vi "Get Result.vi"(8 "error in (no error)":errorcluster, 11 "LUnit Test Case V2 In":refnum<class "LUnit Test Case V2.lvclass">) -> (0 "error out":errorcluster, 2 "Cluster of class private data":T1, 3 "LUnit Test Case V2 Out":refnum<class "LUnit Test Case V2.lvclass">)   [LabVIEW 2020, in "LUnit Test Case V2.lvclass"]
uses:
  LUnit Test Case V2.lvclass
  Framework/Result Types/Assertion Result/Public/TypeDefs/Status.ctl
  Framework/Result Types/Assertion Result/Assertion Result.lvlib
  Framework/Result Types/Assertion Result/Public/TypeDefs/Assertion Type.ctl
  Framework/Result Types/Assertion Result/Assertion Result.ctl
  Framework/Result Types/Method Result/Method Result.ctl
  Framework/Result Types/Method Result/Method Result.lvlib
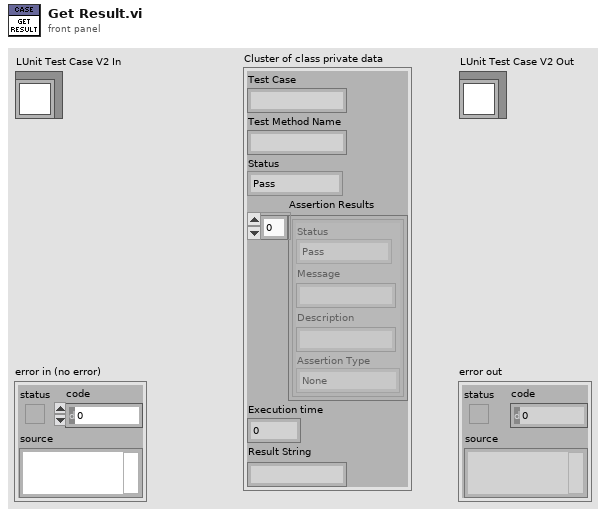
[diagram p1: front panel]
types:
  T1 = typedef "Method Result.lvlib/Method Result.ctl" = cluster{"Test Case":string, "Test Method Name":string, "Status":T2, "Assertion Results":T3[], "Execution time":dbl, "Result String":string}
  T2 = typedef "Assertion Result.lvlib/Status.ctl" = enum16{"Pass", "Fail", "Error", "Skipped", "Setup Error", "Broken", "Teardown Error"}
  T3 = typedef "Assertion Result.lvlib/Assertion Result.ctl" = cluster{"Status":T2, "Message":string, "Description":string, "Assertion Type":T4}
  T4 = typedef "Assertion Result.lvlib/Assertion Type.ctl" = enum16{"None", "Pass", "Fail", "Skip", "Pass if Equal", "Fail if Equal", "Pass if Error", "Fail if Error", "Pass if", "Fail if"}
  T5 = typedef "Result.lvlib/Result.ctl" = cluster{"Case":string, "Method":string, "Message":string, "Description":string, "Status":T6, "Result Type":T7}
  T6 = typedef "Result.lvlib/Status.ctl" = enum16{"Pass", "Fail", "Error", "Skipped", "Setup Error", "Broken", "Teardown Error"}
  T7 = typedef "Result.lvlib/Type.ctl" = enum16{"None", "Pass", "Fail", "Skip", "Pass if Equal", "Fail if Equal", "Pass if Error", "Fail if Error", "Pass if", "Fail if"}
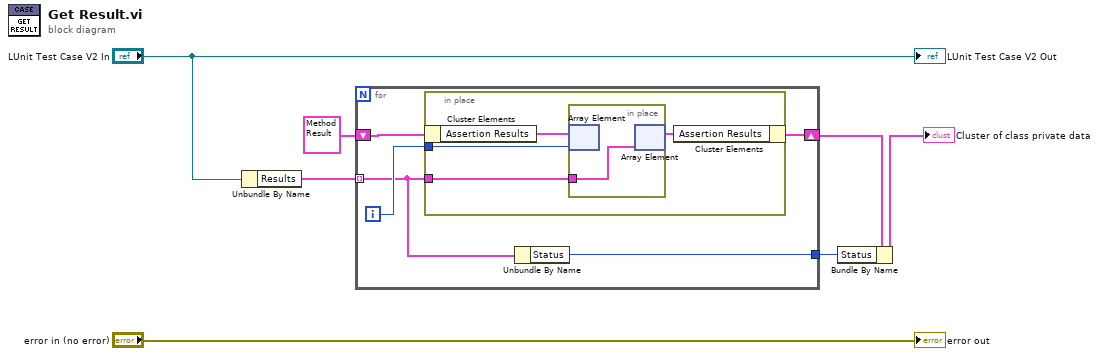
[diagram p0: block diagram]
diagram:
  n1 = Unbundle By Name("LUnit Test Case V2 In") -> ("Results"=w5:T5[])
  n2 = for {
    tunnel: w5 -> [w9] mode=indexing
    shift-right: [w10] -> w3
    shift-left: T1 {"Test Case"="", "Test Method Name"="", "Status"=enum."Pass", "Assertion Results"=[{"Status"=enum."Fail", "Message"="", "Description"="", "Assertion Type"=enum."None"}], "Execution time"=0.0, "Result String"=""} ("Cluster of class private data") -> [w12]
    tunnel: [w8] -> w1
    i -> [w11]
    n3 = in-place {
      in-place-border: w11 -> [w15]
      in-place-border: w9 -> [w14]
      n4 = in-place-cluster #1(w12) -> ("Assertion Results"=w16:T3[])
      n5 = in-place {
        in-place-border: w14 -> [w17]
        n6 = in-place-array #2(w16, w15) -> ()  [unwired: 1 out]
        n7 = in-place-array #2(w17) -> (w13:T3[])  [unwired: 1 out]
      }
      n8 = in-place-cluster #1("Assertion Results"=w13) -> (w10:T1)
    }
    n9 = Unbundle By Name(w9) -> ("Status"=w8:T6)
  }
  n10 = Bundle By Name(cluster=w3, "Status"=w1) -> (→"Cluster of class private data":T1)
  "error out" <- "error in (no error)"
  "LUnit Test Case V2 Out" <- "LUnit Test Case V2 In"
